vi "Set Component Settings.vi"(8 "error in (no error)":errorcluster, 10 "component settings":T1, 11 "Runtime Configuration in":refnum<class "Runtime Configuration.lvclass">) -> (0 "error out":errorcluster, 3 "Runtime Configuration out":refnum<class "Runtime Configuration.lvclass">)   [LabVIEW 2017, in "DSF Core.lvlib" / "Runtime Configuration.lvclass"]
uses:
  Runtime Configuration.lvclass
  Typedefs/DSF Settings Info.ctl
  Typedefs/DSF Version Info.ctl
  Runtime Configuration.lvclass/Runtime Configuration.ctl
  DSF Core.lvlib
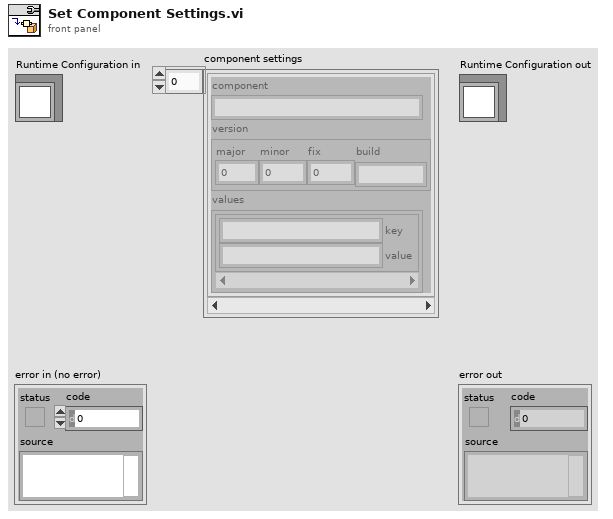
[diagram p1: front panel]
types:
  T1 = typedef "DSF Core.lvlib/DSF Settings Info.ctl" = cluster{"component":string, "version":T2, "values":cluster{"key":string, "value":string}[]}[]
  T2 = typedef "DSF Core.lvlib/DSF Version Info.ctl" = cluster{"major":u32, "minor":u32, "fix":u32, "build":string}
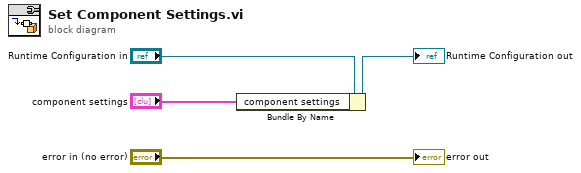
[diagram p0: block diagram]
diagram:
  n1 = Bundle By Name(cluster="Runtime Configuration in", "component settings"="component settings") -> (→"Runtime Configuration out":refnum<class "Runtime Configuration.lvclass">)
  "error out" <- "error in (no error)"
